vi "IndexSampleTimeAreaName.vi"(10 "Row":i32, 11 "SampleInfo列表框":refnum<vi>) -> (2 "Area_name":string, 3 "SampleTime":string)   [LabVIEW 2014, in "ChaxuConfig.lvlib"]
uses:
  ChaxuConfig.lvlib
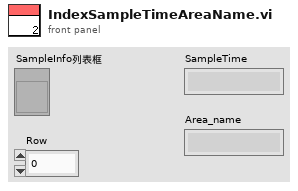
[diagram p1: front panel]
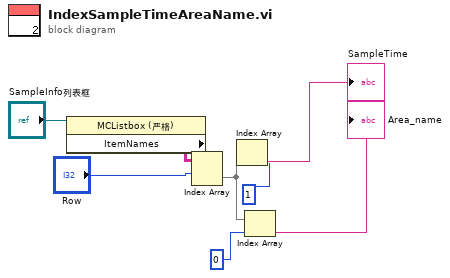
[diagram p0: block diagram]
diagram:
  n1 = property on="属性节点" class="MCListbox (严格)"(reference="SampleInfo列表框") -> ("ItemNames"=w2:string[][])  [unwired: 1 in, 2 out]
  n2 = Index Array(array=w2, index (row)="Row") -> (element=w5:string[])  [unwired: 1 in]
  n3 = Index Array(array=w5, index=1 ("索引")) -> (element=→"SampleTime":string)
  n4 = Index Array(array=w5, index=0) -> (element=→"Area_name":string)
